vi "importAirDelivery.vi"(8 "error in (no error)":errorcluster, 10 "Tuple":T1={"mouse_id"=1217.0, "session_timestamp"="", "timestamp"=0.0, "pulse_time"=0.0}, 11 "Database in":refnum<class "Database.lvclass">) -> (0 "error out":errorcluster, 3 "Database out":refnum<class "Database.lvclass">)   [LabVIEW 2014, in "Database.lvclass"]
uses:
  Database.lvclass
  Database.lvclass/Database.ctl
  <vilib>/addons/database/NI_Database_API.lvlib
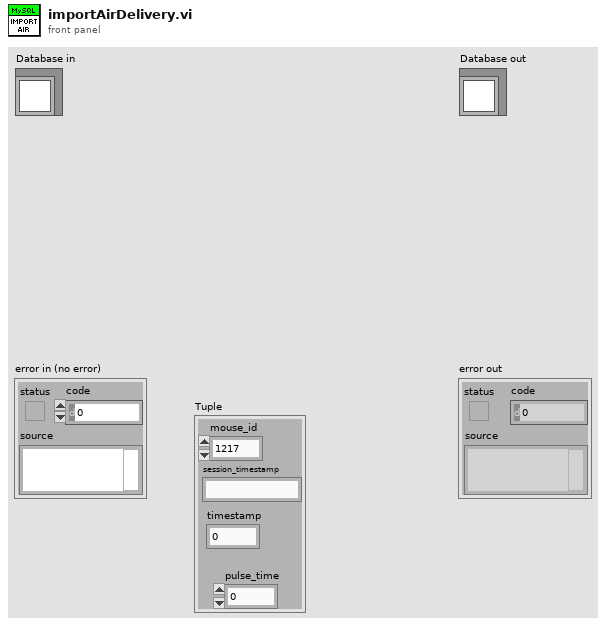
[diagram p1: front panel]
types:
  T1 = cluster{"mouse_id":dbl, "session_timestamp":string, "timestamp":dbl, "pulse_time":dbl}
  T2 = typedef "NI_Database_API.lvlib/Conn ObjectReference.ctl" = refnum<k1>
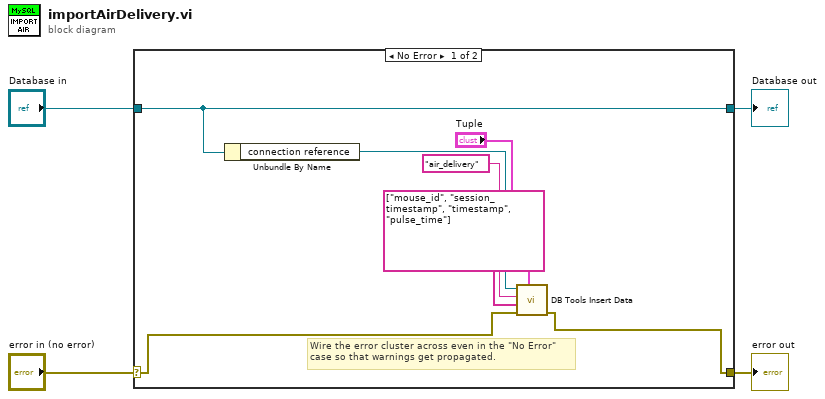
[diagram p0: block diagram]
diagram:
  n1 = case shown="No Error" "error in (no error)" {
    selector: "error in (no error)" -> [w6 w13]
    tunnel: [w5 w13] -> w3
    tunnel: [w7 w12] -> w1
    tunnel: "Database in" -> [w7 w12]
    frame No Error {
      # "Wire the error cluster across even in the \"No Error\"\ncase so that warnings get propagated."
      n2 = Unbundle By Name(w7) -> ("connection reference"=w9:T2)
      n3 = call <vilib>:"DB Tools Insert Data.vi"("data"="Tuple", "error in (no error)"=w6, "columns"=string[] ["mouse_id", "session_timestamp", "timestamp", "pulse_time"], "table"="air_delivery", "connection reference"=w9) -> ("error out"=w5:errorcluster)  [unwired: 5 in, 1 out]
    }
    frame Error {
    }
  }
  "error out" <- w3
  "Database out" <- w1
